vi "Excel_Para.vi"(6 "1_IL,0_uL":bool, 7 "Test parameter":T1, 8 "error in (no error)":errorcluster, 9 "Test?":bool, 10 "Report path in":path, 11 "report in":refnum<class "NI_report.lvclass">) -> (0 "error out":errorcluster, 2 "Report path out":path, 3 "report out":refnum<class "NI_report.lvclass">)   [LabVIEW 2015]
doc: "报表中的电路因子，环境温度，时间常数，温度修正因子"
uses:
  <vilib>/Utility/NIReport.llb/NI_report.lvclass
  <vilib>/addons/_office/_exclsub.llb/font.ctl
  <vilib>/addons/_office/NI_ReportGenerationToolkit.lvlib
panel:
  in  "start(-1,-1)":cluster{"row":i32, "column":i32}
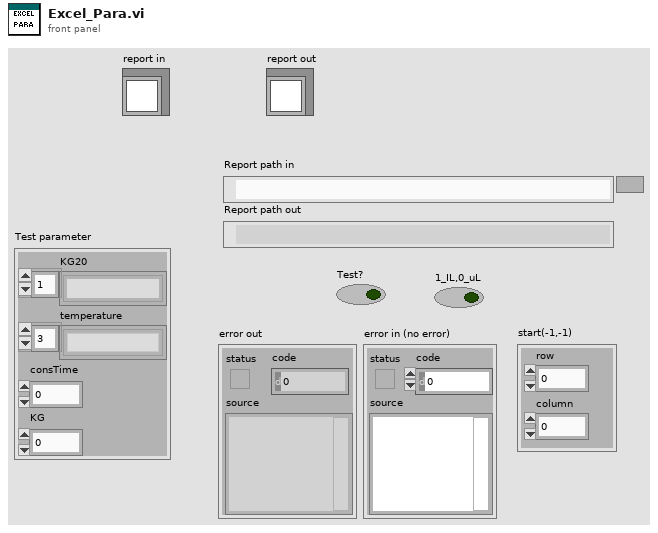
[diagram p1: front panel]
types:
  T1 = cluster{"KG20":string[], "temperature":string[], "consTime":i32, "KG":dbl}
  T2 = typedef "NI_ReportGenerationToolkit.lvlib/font.ctl" = cluster{"font name":string, "font size":dbl, "bold":u16, "italic":u16, "underline":u16, "strike through":u16, "font color":u32}
  T3 = enum16{"maximized", "minimized", "normal", "no change"}
  T4 = enum16{"Standard Report", "HTML", "Word", "Excel"}
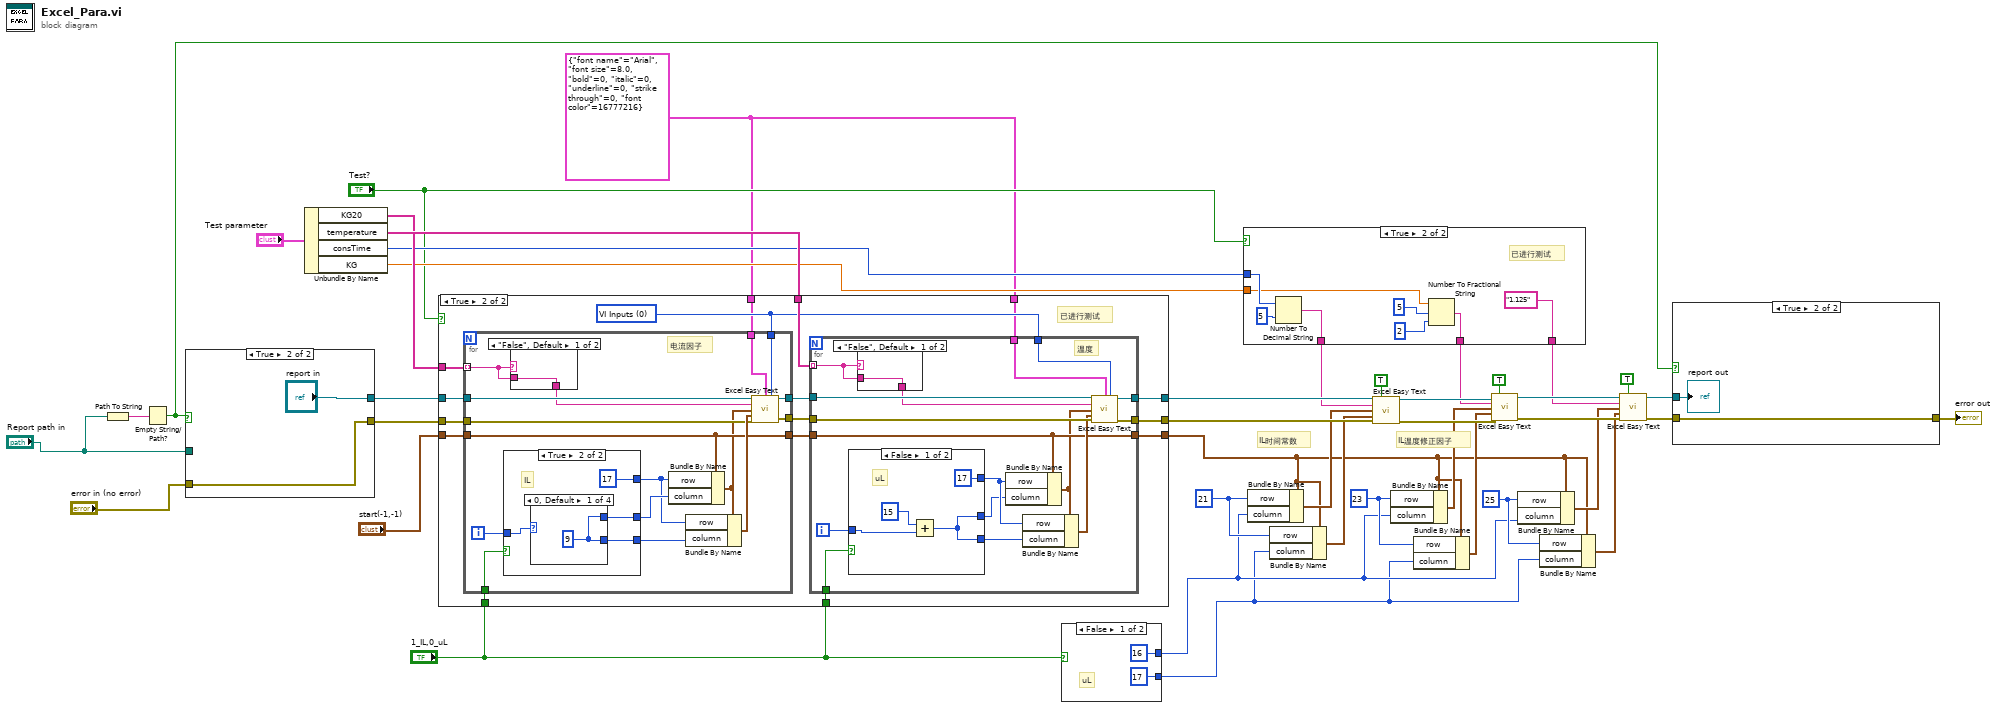
[diagram p0: block diagram]
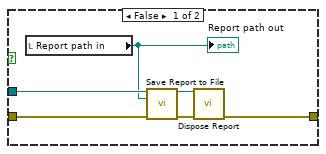
[diagram p2: hidden frame]
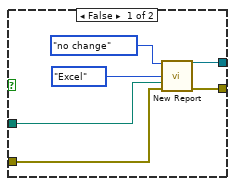
[diagram p3: hidden frame]
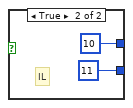
[diagram p4: hidden frame]
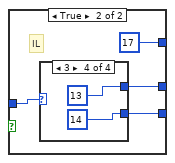
[diagram p6: hidden frame]
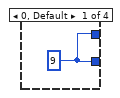
[diagram p7: hidden frame]
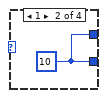
[diagram p8: hidden frame]
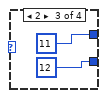
[diagram p9: hidden frame]
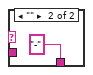
[diagram p10: hidden frame]
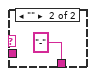
[diagram p11: hidden frame]
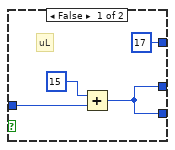
[diagram p12: hidden frame]
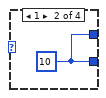
[diagram p13: hidden frame]
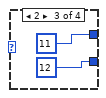
[diagram p14: hidden frame]
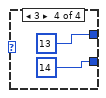
[diagram p15: hidden frame]
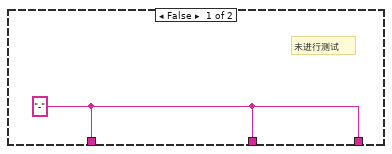
[diagram p16: hidden frame]
diagram:
  w12 = 25 ("row")
  w8 = T2 {"font name"="Arial", "font size"=8.0, "bold"=0, "italic"=0, "underline"=0, "strike through"=0, "font color"=16777216} ("font")
  w33 = 23 ("row")
  w40 = 21 ("row")
  # "IL温度修正因子"
  # "IL时间常数"
  n1 = Path To String(path="Report path in") -> (string=w2:string)
  n2 = Empty String/Path?(string/path=w2) -> (empty?=w1:bool)
  n3 = case shown="True" w1 {
    tunnel: "error in (no error)" -> [w46 w50]
    tunnel: [w45 "report in"] -> w21
    tunnel: [w44 w50] -> w20
    tunnel: "Report path in" -> [w43 _]
    frame False {
      n4 = call <vilib>:"New Report.vi"("window state (normal)"=T3."no change", "report type"=T4."Excel", "template (empty)"=w43, "error in (no error)"=w46) -> ("report out"=w45:refnum<class "NI_report.lvclass">, "error out"=w44:errorcluster)  [unwired: 10 in]
    }
    frame True {
    }
  }
  n5 = Unbundle By Name("Test parameter") -> ("KG20"=w29:string[], "temperature"=w30:string[], "consTime"=w28:i32, "KG"=w26:dbl)
  n6 = case shown="True" "Test?" {
    tunnel: [w53 w67] -> w42
    tunnel: [w52 w66] -> w41
    tunnel: w30 -> [_ w65]
    tunnel: w29 -> [_ w64]
    tunnel: w8 -> [_ w62]
    tunnel: w21 -> [w53 w61]
    tunnel: w20 -> [w52 w60]
    tunnel: "start(-1,-1)" -> [w51 w58]
    tunnel: w8 -> [_ w57]
    tunnel: [w51 w56] -> w7
    tunnel: "1_IL,0_uL" -> [_ w55]
    tunnel: "1_IL,0_uL" -> [_ w54]
    frame False {
      # "未进行测试"
    }
    frame True {
      w63 = u16 0 items=["VI Inputs", "Font Dialog Box"] ("font settings source")
      # "已进行测试"
      n7 = for {
        tunnel: w64 -> [w104] mode=indexing
        tunnel: w58 -> [w106]
        tunnel: [w116] -> w69
        tunnel: [w115] -> w68
        tunnel: w63 -> [w114]
        tunnel: w57 -> [w113]
        tunnel: w61 -> [w112]
        tunnel: w60 -> [w111]
        tunnel: [w106] -> w59
        tunnel: w54 -> [w107]
        i -> [w108]
        # "电流因子"
        n8 = case shown="True" w107 {
          tunnel: [17 ("row") 17 ("row")] -> w102
          tunnel: [w122 w125] -> w109
          tunnel: [w122 w124] -> w110
          tunnel: w108 -> [w123 w126]
          frame False {
            # "uL"
            n9 = Add(x=15, y=w123) -> (x+y=w122:i32)
          }
          frame True {
            # "IL"
            n10 = case shown="0, Default" w126 {
              tunnel: [w128 w129 12 ("row") 14 ("row")] -> w125
              tunnel: [w128 w129 11 ("row") 13 ("row")] -> w124
              frame 0, Default {
                w128 = 9 ("row")
              }
              frame 1 {
                w129 = 10 ("row")
              }
              frame 2 {
              }
              frame 3 {
              }
            }
          }
        }
        n11 = case shown="\"False\", Default" w104 {
          tunnel: [w118 "-"] -> w105
          tunnel: w104 -> [w118 _]
          frame "False", Default {
          }
          frame "" {
          }
        }
        n12 = Bundle By Name(cluster=w106, "row"=w102, "column"=w110) -> (w103:cluster{"row":i32, "column":i32})
        n13 = Bundle By Name(cluster=w103, "row"=w102, "column"=w109) -> (w117:cluster{"row":i32, "column":i32})
        n14 = call <vilib>:"Excel Easy Text.vi"("report in"=w112, "font"=w113, "font settings source"=w114, "text"=w105, "start (-1, -1)"=w103, "end (-1, -1)"=w117, "error in (no error)"=w111) -> ("report out"=w116:refnum<class "NI_report.lvclass">, "error out"=w115:errorcluster)  [unwired: 4 in, 3 out]
      }
      n15 = for {
        tunnel: w69 -> [w85]
        tunnel: w68 -> [w84]
        tunnel: w65 -> [w76] mode=indexing
        tunnel: w59 -> [w78]
        tunnel: [w82] -> w67
        tunnel: [w81] -> w66
        tunnel: w63 -> [w80]
        tunnel: w62 -> [w79]
        tunnel: [w78] -> w56
        tunnel: w55 -> [w73]
        i -> [w74]
        # "温度"
        n16 = case shown="False" w73 {
          tunnel: [17 ("row") 17 ("row")] -> w72
          tunnel: [w89 w92] -> w70
          tunnel: [w89 w91] -> w71
          tunnel: w74 -> [w86 w90]
          frame False {
            # "uL"
            n17 = Add(x=15, y=w86) -> (x+y=w89:i32)
          }
          frame True {
            # "IL"
            n18 = case shown="3" w90 {
              tunnel: [w94 w95 12 ("row") 14 ("row")] -> w92
              tunnel: [w94 w95 11 ("row") 13 ("row")] -> w91
              frame 0, Default {
                w94 = 9 ("row")
              }
              frame 1 {
                w95 = 10 ("row")
              }
              frame 2 {
              }
              frame 3 {
              }
            }
          }
        }
        n19 = case shown="\"False\", Default" w76 {
          tunnel: [w100 "-"] -> w77
          tunnel: w76 -> [w100 _]
          frame "False", Default {
          }
          frame "" {
          }
        }
        n20 = Bundle By Name(cluster=w78, "row"=w72, "column"=w71) -> (w75:cluster{"row":i32, "column":i32})
        n21 = Bundle By Name(cluster=w75, "row"=w72, "column"=w70) -> (w83:cluster{"row":i32, "column":i32})
        n22 = call <vilib>:"Excel Easy Text.vi"("report in"=w85, "font"=w79, "font settings source"=w80, "text"=w77, "start (-1, -1)"=w75, "end (-1, -1)"=w83, "error in (no error)"=w84) -> ("report out"=w82:refnum<class "NI_report.lvclass">, "error out"=w81:errorcluster)  [unwired: 4 in, 3 out]
      }
    }
  }
  n23 = case shown="False" "1_IL,0_uL" {
    tunnel: [16 ("column") 10 ("column")] -> w5
    tunnel: [17 ("column") 11 ("column")] -> w4
    frame False {
      # "uL"
    }
    frame True {
      # "IL"
    }
  }
  n24 = case shown="True" "Test?" {
    tunnel: w28 -> [_ w146]
    tunnel: [w138 w145] -> w27
    tunnel: w26 -> [_ w143]
    tunnel: [w138 w142] -> w25
    tunnel: [w138 "1.125" ("text")] -> w11
    frame False {
      w138 = "-"
      # "未进行测试"
    }
    frame True {
      # "已进行测试"
      n25 = Number To Decimal String(number=w146, width (-)=i16 5) -> (decimal integer string=w145:string)
      n26 = Number To Fractional String(number=w143, width (-)=i16 5, precision (6)=i16 2 ("width (-)")) -> (F-format string=w142:string)  [unwired: 1 in]
    }
  }
  n27 = Bundle By Name(cluster=w7, "row"=w40, "column"=w5) -> (w39:cluster{"row":i32, "column":i32})
  n28 = Bundle By Name(cluster=w7, "row"=w40, "column"=w4) -> (w38:cluster{"row":i32, "column":i32})
  n29 = call <vilib>:"Excel Easy Text.vi"("report in"=w42, "border? (F)"=TRUE, "text"=w27, "start (-1, -1)"=w39, "end (-1, -1)"=w38, "error in (no error)"=w41) -> ("report out"=w37:refnum<class "NI_report.lvclass">, "error out"=w36:errorcluster)  [unwired: 5 in, 3 out]
  n30 = Bundle By Name(cluster=w7, "row"=w33, "column"=w5) -> (w35:cluster{"row":i32, "column":i32})
  n31 = Bundle By Name(cluster=w7, "row"=w33, "column"=w4) -> (w34:cluster{"row":i32, "column":i32})
  n32 = call <vilib>:"Excel Easy Text.vi"("report in"=w37, "border? (F)"=TRUE, "text"=w25, "start (-1, -1)"=w35, "end (-1, -1)"=w34, "error in (no error)"=w36) -> ("report out"=w19:refnum<class "NI_report.lvclass">, "error out"=w18:errorcluster)  [unwired: 5 in, 3 out]
  n33 = Bundle By Name(cluster=w7, "row"=w12, "column"=w5) -> (w14:cluster{"row":i32, "column":i32})
  n34 = Bundle By Name(cluster=w7, "row"=w12, "column"=w4) -> (w13:cluster{"row":i32, "column":i32})
  n35 = call <vilib>:"Excel Easy Text.vi"("report in"=w19, "border? (F)"=TRUE, "text"=w11, "start (-1, -1)"=w14, "end (-1, -1)"=w13, "error in (no error)"=w18) -> ("report out"=w16:refnum<class "NI_report.lvclass">, "error out"=w17:errorcluster)  [unwired: 5 in, 3 out]
  n36 = case shown="True" w1 {
    tunnel: [w150 w154] -> w32
    tunnel: w17 -> [w149 w154]
    tunnel: w16 -> [w148 w153]
    frame False {
      n37 = local read "Report path in"() -> (w147:path)
      "Report path out" <- w147
      n38 = call-dynamic "Save Report to File.vi"("report in"=w148, "report file path"=w147, "error in (no error)"=w149) -> ("report out"=w152:refnum<class "NI_report.lvclass">, "error out"=w151:errorcluster)  [unwired: 11 in]
      n39 = call-dynamic "Dispose Report.vi"("report in"=w152, "error in (no error)"=w151) -> ("error out"=w150:errorcluster)  [unwired: 13 in]
    }
    frame True {
      "report out" <- w153
    }
  }
  "error out" <- w32
